vi "Sub Initialize.vi"(8 "error in (no error)":errorcluster, 11 "Channel Scanner in":refnum<class "Channel Scanner.lvclass">) -> (0 "error out":errorcluster, 2 "Initialize Result":refnum<class "Acquired Result.lvclass">, 3 "Channel Scanner out":refnum<class "Channel Scanner.lvclass">)   [LabVIEW 2016, in "Channel Scanner.lvclass"]
uses:
  Channel Scanner.lvclass
  C:/Program Files/National Instruments/LabVIEW 2016/vi.lib/ActorFramework/Actor/Actor.lvclass
  Measure_core/Results/Acquired Result/Acquired Result.lvclass
  NHMFL_Core/Libraries/Instruments/Instrument Driver/Channel Scanner Driver/Channel Scanner Driver.lvclass/Channel Scanner Driver.ctl
  <vilib>/ActorFramework/Actor/Actor.lvclass/Actor.ctl
  <vilib>/ActorFramework/Message Enqueuer/Message Enqueuer.lvclass/Message Enqueuer.ctl
  Measure_core/Da Base Messages/Subscribe Request Msg/Subscribe Request Msg.lvclass/Subscribe Request Msg.ctl
  Channel Scanner.lvclass/Channel Scanner.ctl
  NHMFL_Core/Libraries/Instruments/Instrument Driver/Channel Scanner Driver/Write Next channel idx.vi
  NHMFL_Core/Libraries/Instruments/Instrument Driver/Channel Scanner Driver/Write Scan Channels.vi
  <vilib>/ActorFramework/Message Enqueuer/Init from Existing Queue.vi
  <vilib>/ActorFramework/Message Enqueuer/Enqueue.vi
  Measure_core/Da Base Messages/Subscribe Request Msg/Subscribe Request Msg.lvclass
  C:/Program Files/National Instruments/LabVIEW 2016/vi.lib/ActorFramework/Message/Message.lvclass
  Read Scanner driver.vi
  Read Channel scanner configuration.vi
  Write Scanner driver.vi
  <vilib>/ActorFramework/Message Priority Queue/Priority Enqueue.vi
  NHMFL_Core/Libraries/Instruments/Instrument Driver/Channel Scanner Driver/Channel Scanner Driver.lvclass
  <vilib>/ActorFramework/Message Enqueuer/Message Enqueuer.lvclass
  Measure_core/Instrument Recorders/Instrument Recorder/Instrument Recorder.lvclass
  <vilib>/ActorFramework/Actor/Actor.lvclass
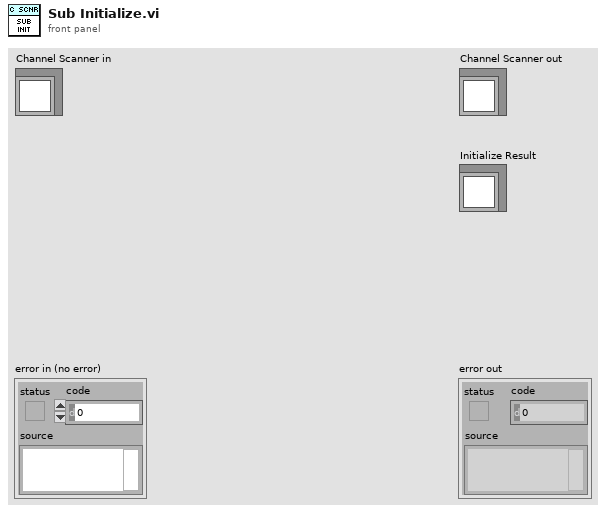
[diagram p1: front panel]
types:
  T1 = typedef "Channel Scanner Configuration.ctl" = cluster{"Scan channels":i32[], "Group with measurement":string}
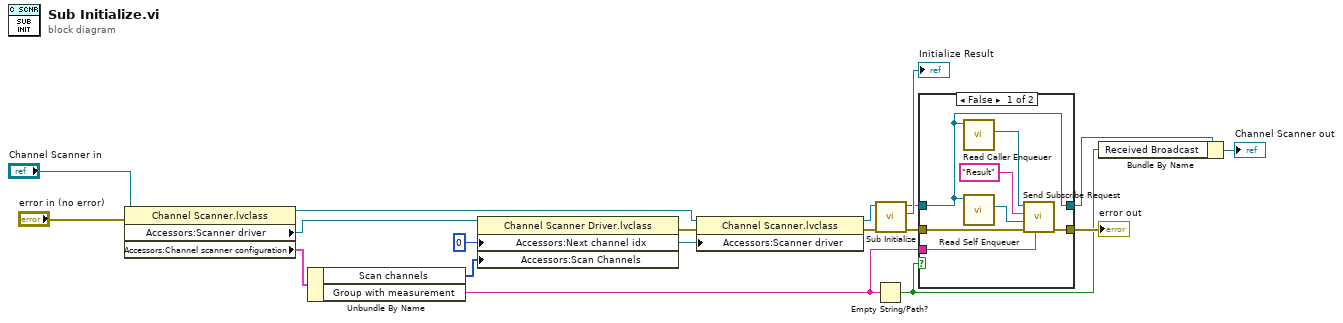
[diagram p0: block diagram]
diagram:
  n1 = property class="Channel Scanner.lvclass"(reference="Channel Scanner in", error in="error in (no error)") -> (reference out=w11:refnum<class "Channel Scanner.lvclass">, "Accessors:Scanner driver"=w17:refnum<class "Channel Scanner Driver.lvclass">, "Accessors:Channel scanner configuration"=w15:T1)  [unwired: 1 out]
  n2 = Unbundle By Name(w15) -> ("Scan channels"=w14:i32[], "Group with measurement"=w7:string)
  n3 = property class="Channel Scanner Driver.lvclass"(reference=w17, "Accessors:Next channel idx"=0 ("Next channel idx"), "Accessors:Scan Channels"=w14) -> (reference out=w12:refnum<class "Channel Scanner Driver.lvclass">, error out=w13:errorcluster)  [unwired: 1 in]
  n4 = property class="Channel Scanner.lvclass"(reference=w11, error in=w13, "Accessors:Scanner driver"=w12) -> (reference out=w9:refnum<class "Channel Scanner.lvclass">, error out=w10:errorcluster)
  n5 = Empty String/Path?(string/path=w7) -> (empty?=w1:bool)
  n6 = call-parent "Sub Initialize.vi"("error in (no error)"=w10, "Instrument Recorder in"=w9) -> ("error out"=w4:errorcluster, "Initialize Result"=→"Initialize Result":refnum<class "Acquired Result.lvclass">, "Instrument Recorder out"=w6:refnum<class "Channel Scanner.lvclass">)  [unwired: 7 in]
  n7 = case shown="False" w1 {
    tunnel: w7 -> [w24 _]
    tunnel: w6 -> [w21 w28]
    tunnel: [w21 w28] -> w5
    tunnel: w4 -> [w26 w27]
    tunnel: [w25 w27] -> w3
    frame False {
      n8 = call <vilib>:"Read Caller Enqueuer.vi"("Actor"=w21) -> ("Caller Enqueuer"=w22:refnum<class "Message Enqueuer.lvclass">)  [unwired: 10 in]
      n9 = call <vilib>:"Read Self Enqueuer.vi"("Actor"=w21) -> ("Self Enqueuer"=w20:refnum<class "Message Enqueuer.lvclass">)  [unwired: 10 in]
      n10 = call "Send Subscribe Request.vi"("Broadcaster"=w24, "error in (no error)"=w26, "Subscriber Enqueuer"=w20, "Topic"="Result", "Message Enqueuer"=w22) -> ("error out"=w25:errorcluster)  [unwired: 5 in, 1 out]
    }
    frame True {
    }
  }
  "error out" <- w3
  n11 = Bundle By Name(cluster=w5, "Received Broadcast"=w1) -> (→"Channel Scanner out":refnum<class "Channel Scanner.lvclass">)
